vi "Read Thrust Loss.vi"(8 "error in (no error)":errorcluster, 11 "Thrust Allocation in":refnum<class "Thrust Allocation.lvclass">) -> (0 "error out":errorcluster, 2 "Thrust Loss":dbl[](array[numeric]), 3 "Thrust Allocation out":refnum<class "Thrust Allocation.lvclass">)   [LabVIEW 2011]
uses:
  Thrust Allocation.lvclass
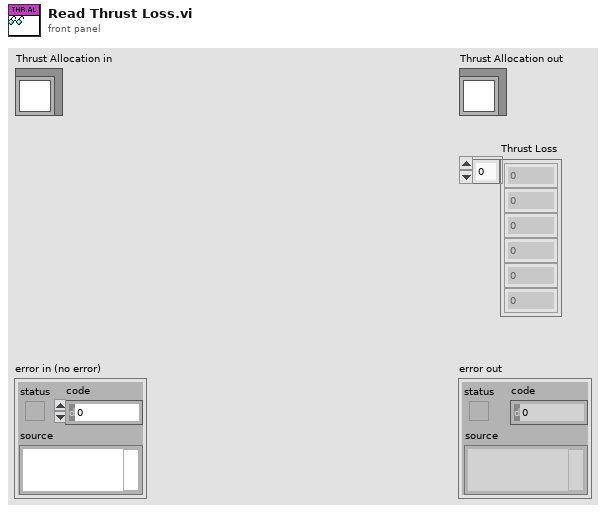
[diagram p1: front panel]
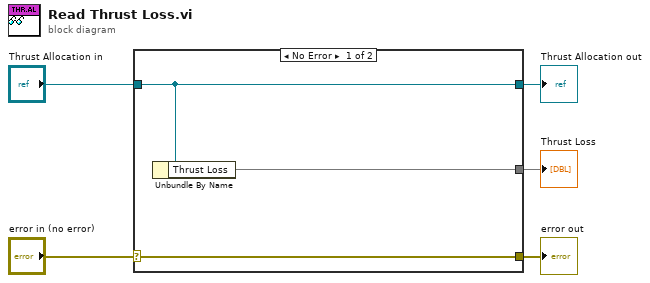
[diagram p0: block diagram]
diagram:
  n1 = case shown="No Error" "error in (no error)" {
    selector: "error in (no error)" -> [w8 w9]
    tunnel: [w8 w9] -> w4
    tunnel: [w7 w10] -> w2
    tunnel: "Thrust Allocation in" -> [w7 w10]
    tunnel: [w6 _] -> w1
    frame No Error {
      n2 = Unbundle By Name(w7) -> ("Thrust Loss"=w6)
    }
    frame Error {
    }
  }
  "error out" <- w4
  "Thrust Allocation out" <- w2
  "Thrust Loss" <- w1
